vi "Shooter.vi"(8 "error in":errorcluster, 9 "Override?":bool, 10 "Override Setpoint":dbl, 11 "Load Ball Finished":bool) -> (0 "error out":errorcluster, 1 "Shooter Operation":T1(ring), 2 "Finished":bool, 3 "Load Ball":bool)   [LabVIEW 2015]
uses:
  <vilib>/Rock Robotics/WPI/CAN/TalonSRX/WPI_CANTalonSRX_APIControlMode.ctl
  <vilib>/Rock Robotics/Network Tables/NT Read Boolean.vi
  Robot Global Data.vi
  Team900-VIs/navX Library v2/navX Library v2.lvlib
panel:
  in  "Idle Speed":dbl=40.0 format="%#_13g"
  out "Shooter Speed (ticks per 100 ms)":dbl(graph)
  in  "Finished? (aim)":bool
  in  "Yaw":dbl
  out "SetSpeed":dbl
  in  "Goal Distance":dbl
  in  "Goal Angle":dbl
  in  "Goal Detected":bool
  in  "Distance to Motor Speed Conversions (Feet to ticks/100ms)":dbl[](array[numeric])=[250.0, 240.0, 210.0, 203.0, 193.0, 187.0, 192.0, 195.0, 197.0, 199.35, 201.73, 208.0]
  in  "Shooter Operation-Test Mode":T1(ring)
  in  "Encoder Velocity":dbl
  out "Turret Angle":T2(graph)
  in  "Setpoint":dbl format="%#_13g"
  in  "Speed Setpoint":dbl=220.0 format="%#_13g"
  in  "Max Shooter Speed (Rpm)":dbl=220.0
  in  "Turret revolutions per shooter revolution":dbl=15.0
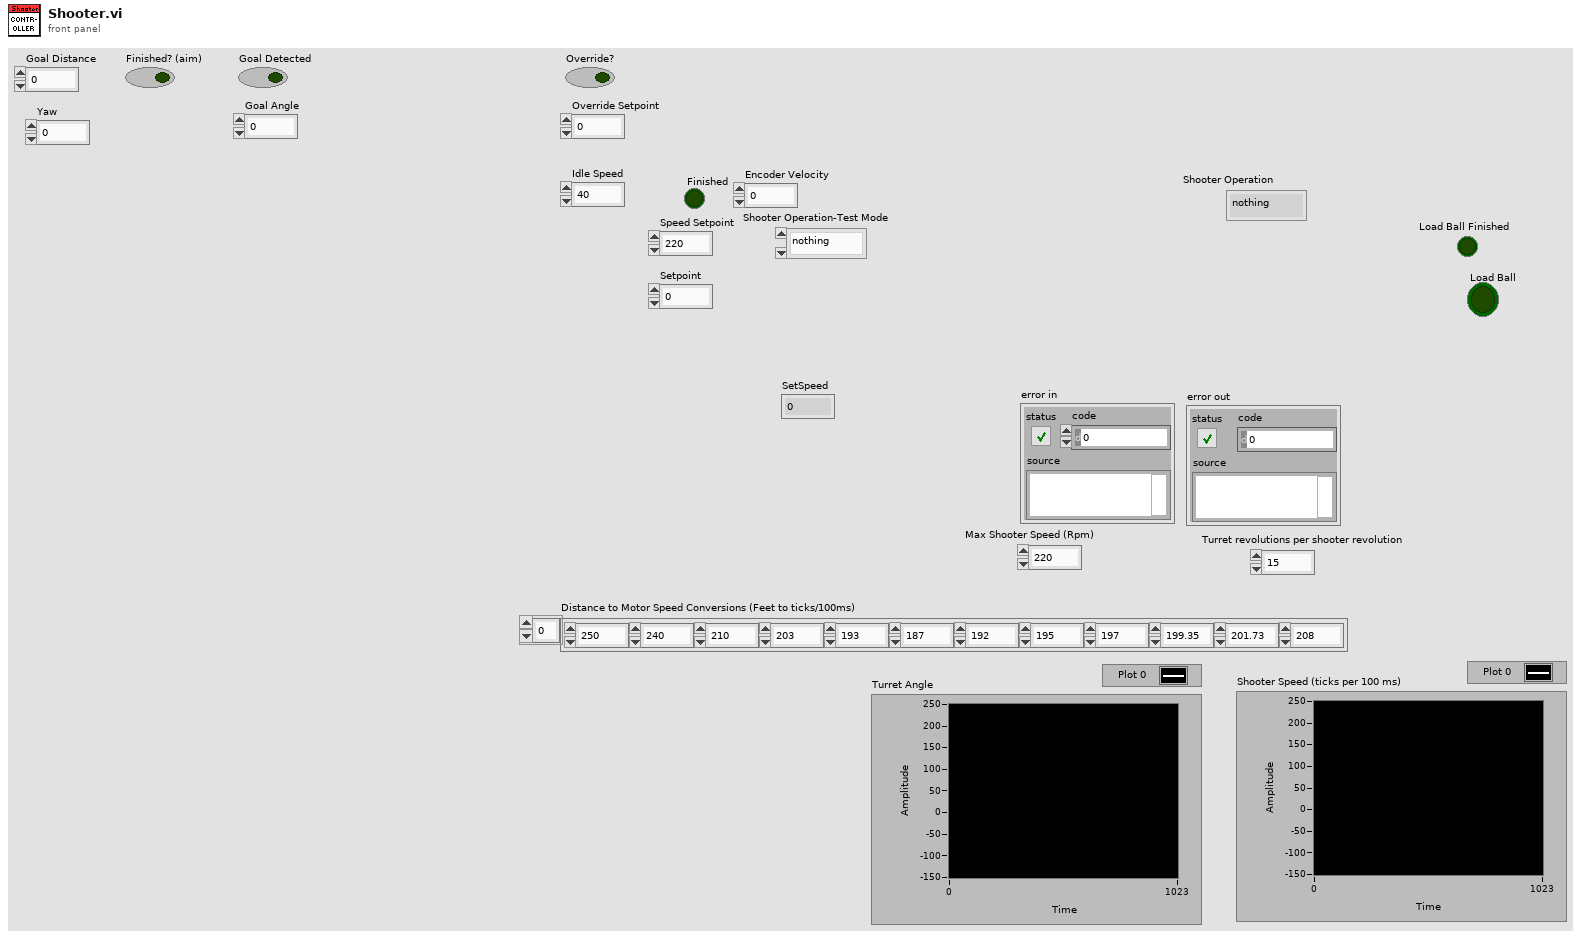
[diagram p1: front panel]
types:
  T1 = enum16{"nothing", "Fire", "Aim Goal", "Aim Foward"}
  T2 = cluster{"[0]":dbl, "[1]":dbl, "[2]":dbl, "[3]":dbl, "[4]":dbl, "[5]":dbl, "[6]":dbl, "[7]":dbl, "[8]":dbl}
  T3 = typedef "navX Library v2.lvlib/Z900_navX_DeviceTypeDef.ctl" = cluster{"Interface":cluster{"Protocol":T4, "Update Rate (4Hz-60Hz)":u8, "navX Open TypeDef":variant}, "Notify Packet":refnum<notifier>, "Loop VI Refnum":refnum<vi>, "Ready to Close Occurrence Refnum":refnum<k4>}
  T4 = typedef "navX Library v2.lvlib/Z900_navX_ProtocolTypeDef.ctl" = enum16{"SERIAL", "I2C", "SPI"}
  T5 = typedef "WPI_CANTalonSRX_APIControlMode.ctl" = enum8{"Percent VBus", "Speed", "Position", "Slave", "Unchanged / Invalid", "Voltage Compensation", "Current", "Motion Profile"}
  T6 = cluster{"Yaw":dbl, "Roll":dbl, "Pitch":dbl, "Heading":dbl, "Fused Heading":dbl}
  T7 = typedef "WPI_MotorControlDeviceRef.ctl" = cluster{"DeviceStatus":errorcluster, "Type":T8, "PWM":cluster{"PWM Channel":T9, "DeadBand":T10}, "CAN":cluster{"Device Number":u8, "Control Mode":T11, "Semaphore":T12, "Max Vout":dbl, "TalonSRX Control Mode":T5}, "Invert":bool}
  T8 = typedef "WPI_MotorControlType.ctl" = enum16{"PWM", "CAN", "CANTalonSRX"}
  T9 = typedef "FPGA_DIOPWMChannel.ctl" = enum8{"PWM 0", "PWM 1", "PWM 2", "PWM 3", "PWM 4", "PWM 5", "PWM 6", "PWM 7", "PWM 8", "PWM 9", "PWM MXP 0", "PWM MXP 1", "PWM MXP 2", "PWM MXP 3", "PWM MXP 4", "PWM MXP 5", "PWM MXP 6", "PWM MXP 7", "PWM MXP 8", "PWM MXP 9", "Invalid"}
  T10 = typedef "WPI_PWMDeadband.ctl" = cluster{"Name":string, "maxPositivePwm":i32, "minPositivePwm":i32, "centerPwm":i32, "maxNegativePwm":i32, "minNegativePwm":i32, "angularRange":u16}
  T11 = typedef "WPI_CANJaguar_ControlMode.ctl" = enum8{"Percent VBus", "Current", "Speed", "Position", "Voltage"}
  T12 = typedef "Semaphore RefNum" = refnum<k1>
  T13 = typedef "WPI_CANTalonSRX_GlobalStatus.ctl" = cluster{"Applied Throttle":dbl, "Module Enabled":bool, "CAN Error":errorcluster, "Closed Loop Error":dbl, "Forward Limit Switch Closed":bool, "Reverse Limit Switch Closed":bool, "Sensor Position":dbl, "Sensor Velocity":dbl, "Current":dbl, "Sticky Fault - Over Temp":bool, "Sticky Fault - Under Voltage":bool, "Sticky Fault - Forward Limit":bool, "Sticky Fault - Reverse Limit":bool, "Sticky Fault - Forward Soft Limit":bool, "Sticky Fault - Reverse Soft Limit":bool, "Brake is Enabled":bool, "Encoder Position":dbl, "Encoder Velocity":dbl, "Encoder Index Count":dbl, "Encoder A Pin State":bool, "Encoder B Pin State":bool, "Encoder Index Pin State":bool, "Analog In":dbl, "Analog In Velocity":dbl, "Temperature (C)":dbl, "Battery Voltage":dbl, "Control 5 Is Supported":bool, "Current Profile Slot Select":dbl, "Pos Div 8":bool, "Vel Div 4":bool, "Pulse Width Position":i32, "Pulse Width Velocity":i32, "Pulse Width Rise To Rise (us)":i32, "Pulse Width Rise To Fall (us)":i32, "Mot Prof Active Is Under Run":bool, "Mot Prof Active Has Under Run":bool, "Mot Prof Active Is Last":bool, "Mot Prof Active Velocity Only":bool, "Mot Prof Active Is Valid":bool, "Mot Prof Buffer Is Full":bool, "Mot Prof Active Profile Slot Select":i32, "Mot Prof NextID":i32, "Mot Prof Count":i32, "Mot Prof Active Velocity":dbl, "Mot Prof Active Position":dbl, "Mot Prof Output Enable":i32}
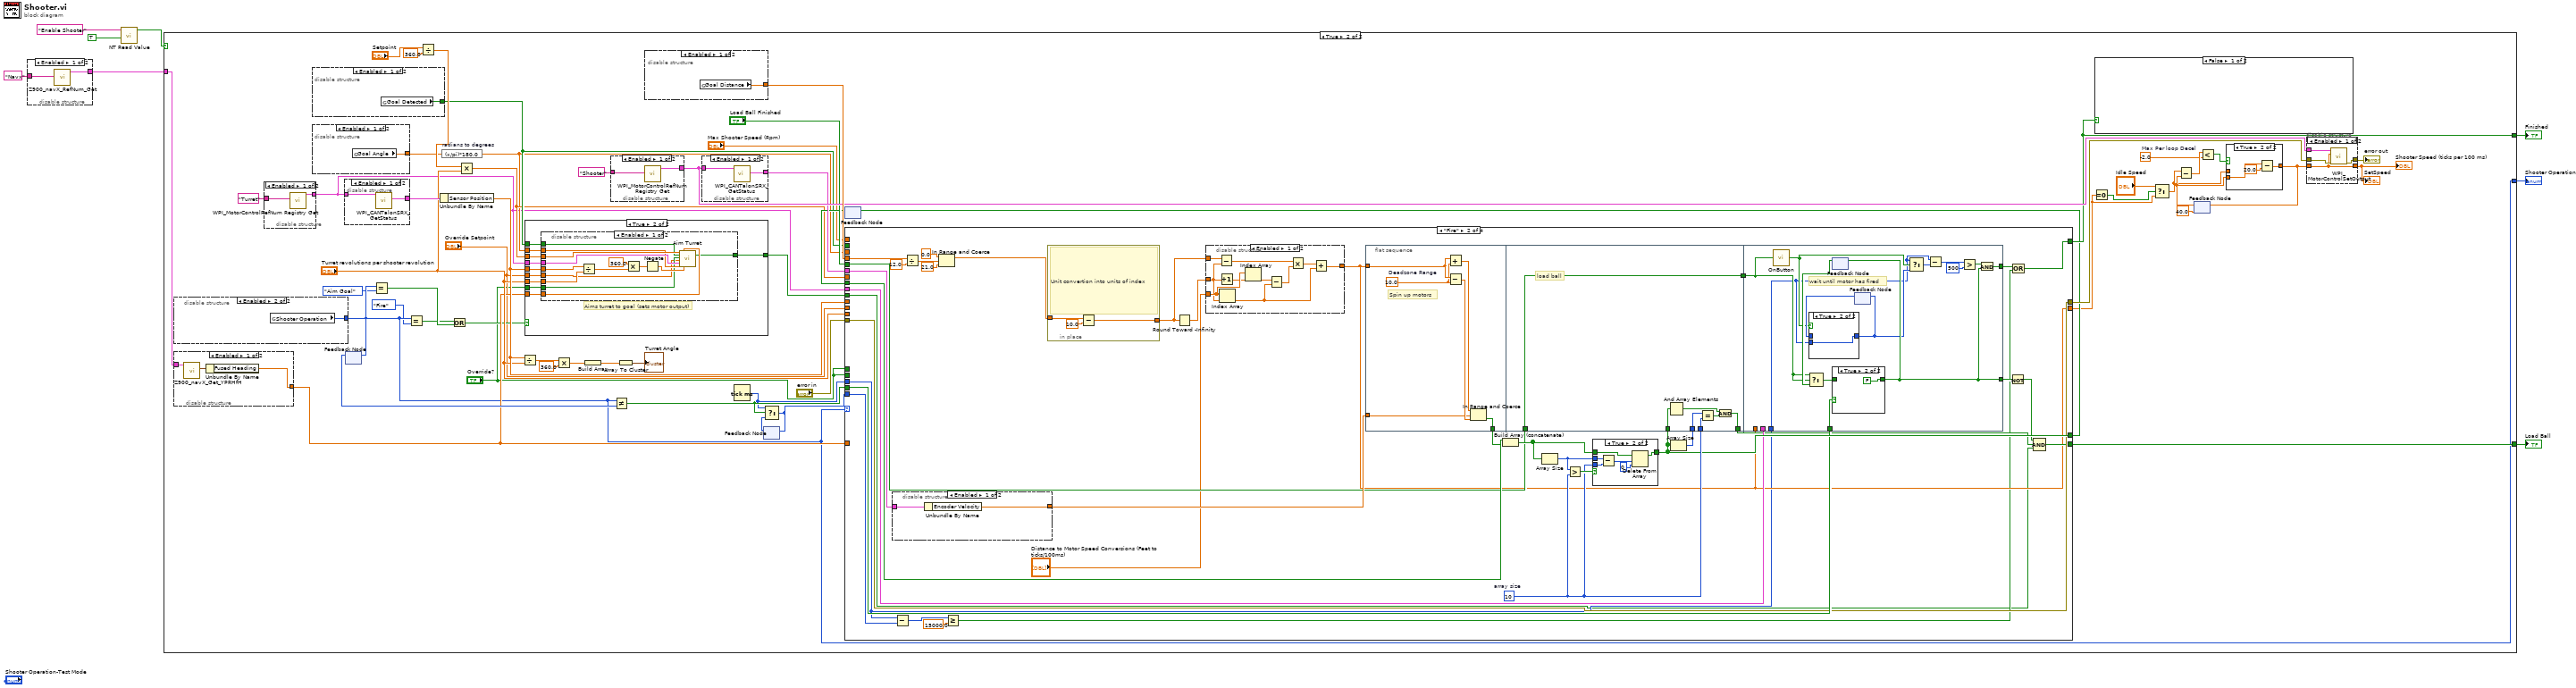
[diagram p0: block diagram]
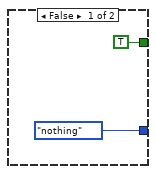
[diagram p3: hidden frame]
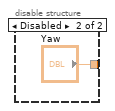
[diagram p5: hidden frame]
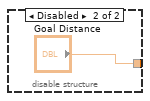
[diagram p6: hidden frame]
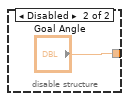
[diagram p7: hidden frame]
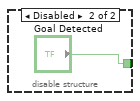
[diagram p8: hidden frame]
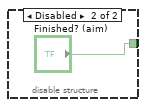
[diagram p10: hidden frame]
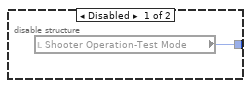
[diagram p11: hidden frame]
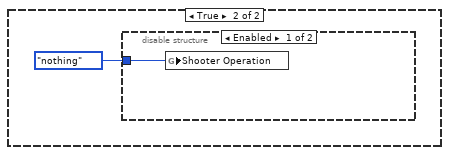
[diagram p17: hidden frame]
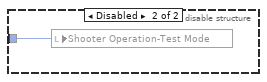
[diagram p18: hidden frame]
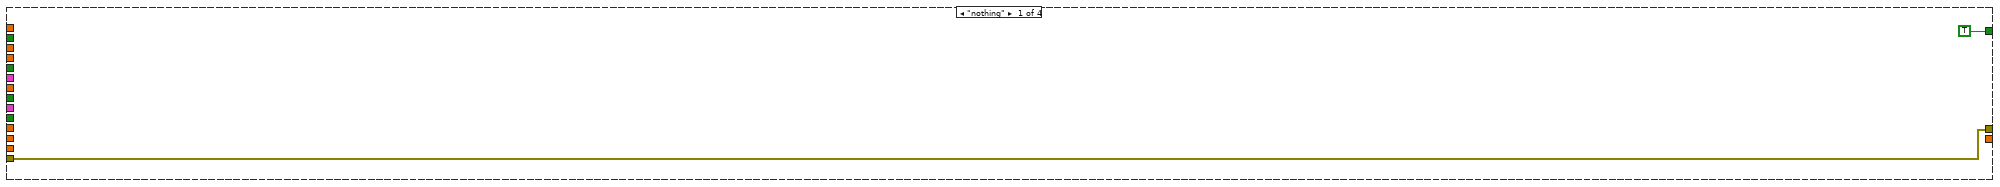
[diagram p19: hidden frame]
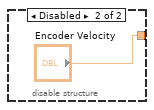
[diagram p20: hidden frame]
diagram:
  n1 = disable-structure shown="Enabled" {
    disable-tunnel: "Navx" ("refnum name") -> [w10 _]
    disable-tunnel: [w9 _] -> w1
    frame Enabled {
      n2 = call "Z900_navX_RefNum_Get.vi"("refnum name"=w10) -> ("navX Device"=w9:T3)  [unwired: 9 in, 1 out]
    }
    frame Disabled {
    }
  }
  n3 = call-poly <vilib>:"NT Read Value.vi"("Default Value"=TRUE, "Name"="Enable Shooter") -> ("Boolean"=w5:bool)  [unwired: 8 in, 1 out]
  n4 = case shown="True" w5 {
    tunnel: [_ w57] -> w6
    tunnel: [T1."nothing" ("Shooter Operation") w27] -> w8
    tunnel: [TRUE w55] -> w7
    tunnel: w1 -> [_ w41]
    frame False {
    }
    frame True {
      w21 = -2.0  # Max Per loop Decel
      n5 = disable-structure shown="Enabled" {
        disable-tunnel: [w109 w110] -> w27
        frame Disabled {
          n6 = local read "Shooter Operation-Test Mode"() -> (w109:T1)
        }
        frame Enabled {
          n7 = global read "Robot Global Data.vi" "Shooter Operation"() -> (w110:T1)
        }
      }
      n8 = disable-structure shown="Enabled" {
        disable-tunnel: w41 -> [w76 _]
        disable-tunnel: [w74 "Yaw"] -> w34
        frame Enabled {
          n9 = call "Z900_navX_Get_YPRHfH.vi"("navX Device"=w76) -> ("YRPHfH"=w75:T6)  [unwired: 7 in, 3 out]
          n10 = Unbundle By Name(w75) -> ("Fused Heading"=w74:dbl)
        }
        frame Disabled {
        }
      }
      n11 = disable-structure shown="Enabled" {
        disable-tunnel: "Turret" ("refnum name") -> [w116 _]
        disable-tunnel: [w115 _] -> w31
        frame Enabled {
          n12 = call <vilib>:"WPI_MotorControlRefNum Registry Get.vi"("refnum name"=w116) -> ("MotorControlDevRef"=w115:T7)  [unwired: 9 in, 1 out]
        }
        frame Disabled {
        }
      }
      n13 = disable-structure shown="Enabled" {
        disable-tunnel: [w82 "Goal Detected"] -> w42
        frame Enabled {
          n14 = global read "Robot Global Data.vi" "Goal Detected"() -> (w82:bool)
        }
        frame Disabled {
        }
      }
      n15 = disable-structure shown="Enabled" {
        disable-tunnel: [w80 "Goal Angle"] -> w23
        frame Enabled {
          n16 = global read "Robot Global Data.vi" "Goal Angle"() -> (w80:dbl)
        }
        frame Disabled {
        }
      }
      n17 = disable-structure shown="Enabled" {
        disable-tunnel: [w112 _] -> w51
        disable-tunnel: w31 -> [w111 _]
        frame Enabled {
          n18 = call <vilib>:"WPI_CANTalonSRX_GetStatus.vi"("CAN Talon SRX Ref"=w111) -> ("Talon SRX Status"=w112:T13)  [unwired: 8 in, 2 out]
        }
        frame Disabled {
        }
      }
      n19 = feedback #1() -> (w66:T1)  [unwired: 1 in]
      n20 = feedback-in #1(w27) -> ()
      n21 = Equal?(x=w27, y=T1."Aim Goal") -> (x = y?=w29:bool)
      n22 = Equal?(x=w27, y=T1."Fire") -> (x = y?=w28:bool)
      n23 = Divide(x="Setpoint", y=360.0) -> (x/y=w46:dbl)
      n24 = Unbundle By Name(w51) -> ("Sensor Position"=w36:dbl)
      n25 = expression code="(x/pi)*180.0" "radians to degrees"(w23) -> (w32:dbl)
      n26 = Or(x=w28, y=w29) -> (x .or. y?=w24:bool)
      n27 = Multiply(x=w46, y="Turret revolutions per shooter revolution") -> (x*y=w33:dbl)
      n28 = Divide(x=w36, y="Turret revolutions per shooter revolution") -> (x/y=w48:dbl)
      n29 = case shown="True" w24 {
        tunnel: w36 -> [_ w93]
        tunnel: "Turret revolutions per shooter revolution" -> [_ w92]
        tunnel: w34 -> [_ w91]
        tunnel: w33 -> [_ w90]
        tunnel: w32 -> [_ w89]
        tunnel: w31 -> [_ w88]
        tunnel: w42 -> [_ w87]
        tunnel: [_ w86] -> w30
        tunnel: "Override?" -> [_ w85]
        tunnel: "Override Setpoint" -> [_ w84]
        frame False {
        }
        frame True {
          # "Aims turret to goal (sets motor output)"
          n30 = disable-structure shown="Enabled" {
            disable-tunnel: w93 -> [w104 _]
            disable-tunnel: w92 -> [w103 _]
            disable-tunnel: w91 -> [w102 _]
            disable-tunnel: w90 -> [w101 _]
            disable-tunnel: w89 -> [w98 _]
            disable-tunnel: w88 -> [w99 _]
            disable-tunnel: w87 -> [w100 _]
            disable-tunnel: [w96 "Finished? (aim)"] -> w86
            disable-tunnel: w85 -> [w95 _]
            disable-tunnel: w84 -> [w94 _]
            frame Enabled {
              n31 = Divide(x=w104, y=w103) -> (x/y=w107:dbl)
              n32 = Multiply(x=360.0, y=w107) -> (x*y=w106:dbl)
              n33 = Negate(x=w106) -> (-x=w97:dbl)
              n34 = call "Aim Turret.vi"("Setpoint (testing purposes only)"=w101, "Goal Detected"=w100, "Override?"=w95, "Override Setpoint"=w94, "MotorControlDevRef"=w99, "Goal Angle Degrees 0=straight ahead"=w98, "Yaw (degrees 0 = straight ahead gets larger clockwise)"=w102, "Sensor Position (degrees)"=w97) -> ("Finished?"=w96:bool)  [unwired: 10 in, 1 out]
            }
            frame Disabled {
            }
          }
        }
      }
      n35 = Multiply(x=w48, y=360.0) -> (x*y=w44:dbl)
      n36 = Build Array(w44) -> (w50:dbl[])
      n37 = disable-structure shown="Enabled" {
        disable-tunnel: "Shooter" ("refnum name") -> [w118 _]
        disable-tunnel: [w117 _] -> w61
        frame Enabled {
          n38 = call <vilib>:"WPI_MotorControlRefNum Registry Get.vi"("refnum name"=w118) -> ("MotorControlDevRef"=w117:T7)  [unwired: 9 in, 1 out]
        }
        frame Disabled {
        }
      }
      n39 = Not Equal?(x=w27, y=w66) -> (x != y?=w52:bool)
      n40 = Array To Cluster(array=w50) -> (cluster=→"Turret Angle":T2)
      n41 = disable-structure shown="Enabled" {
        disable-tunnel: [w78 "Goal Distance"] -> w68
        frame Enabled {
          n42 = global read "Robot Global Data.vi" "Goal Distance"() -> (w78:dbl)
        }
        frame Disabled {
        }
      }
      n43 = disable-structure shown="Enabled" {
        disable-tunnel: w61 -> [w114 _]
        disable-tunnel: [w113 _] -> w58
        frame Enabled {
          n44 = call <vilib>:"WPI_CANTalonSRX_GetStatus.vi"("CAN Talon SRX Ref"=w114) -> ("Talon SRX Status"=w113:T13)  [unwired: 8 in, 2 out]
        }
        frame Disabled {
        }
      }
      n45 = Tick Count (ms)() -> (millisecond timer value=w37:u32)
      n46 = feedback #2() -> (w65:u32)  [unwired: 1 in]
      n47 = Select(t=w37, s=w52, f=w65) -> (s? t:f=w64:u32)
      n48 = feedback-in #2(w64) -> ()
      n49 = feedback #3() -> (w54:bool[])  [unwired: 1 in]
      n50 = case shown="\"Fire\"" w27 {
        tunnel: [TRUE w156 w222 w227] -> w55
        tunnel: w32 -> [_ _ _ _]
        tunnel: w68 -> [_ w134 _ _]
        tunnel: [_ w140 _ _] -> w40
        tunnel: w58 -> [_ w166 _ _]
        tunnel: w54 -> [_ w163 _ _]
        tunnel: "error in" -> [w129 w149 w223 w231]
        tunnel: w42 -> [_ _ _ _]
        tunnel: w31 -> [_ w146 _ w232]
        tunnel: "Max Shooter Speed (Rpm)" -> [_ _ _ _]
        tunnel: w34 -> [_ _ _ _]
        tunnel: w64 -> [_ w153 _ _]
        tunnel: [w129 w149 w223 w238] -> w60
        tunnel: [_ w143 _ _] -> w57
        tunnel: "Load Ball Finished" -> [_ w148 _ _]
        tunnel: [_ w152 _ _] -> w53
        tunnel: w37 -> [_ w138 _ _]
        tunnel: w52 -> [_ w150 _ _]
        tunnel: w33 -> [_ _ _ w237]
        tunnel: "Turret revolutions per shooter revolution" -> [_ _ _ w229]
        tunnel: w36 -> [_ _ _ w230]
        tunnel: w30 -> [_ w135 w222 _]
        tunnel: "Override Setpoint" -> [_ _ _ w226]
        tunnel: "Override?" -> [_ _ _ w225]
        tunnel: "Override?" -> [_ _ _ w224]
        frame "nothing" {
        }
        frame "Fire" {
          w158 = 10  # array size
          n51 = disable-structure shown="Enabled" {
            disable-tunnel: w166 -> [w168 _]
            disable-tunnel: [w167 "Encoder Velocity"] -> w165
            frame Enabled {
              n52 = Unbundle By Name(w168) -> ("Encoder Velocity"=w167:dbl)
            }
            frame Disabled {
            }
          }
          n53 = Subtract(x=w138, y=w153) -> (x-y=w154:u32)
          n54 = Divide(x=w134, y=12.0) -> (x/y=w133:dbl)
          n55 = In Range and Coerce(upper limit=0.0, x=w133, lower limit=21.0) -> (coerced(x)=w130:dbl)  [unwired: 1 out]
          n56 = Greater Or Equal?(x=w154, y=15000.0) -> (x >= y?=w139:bool)
          n57 = in-place {
            in-place-border: [w171] -> w141
            in-place-border: w130 -> [w172]
            # "Unit convertion into units of index"
            n58 = Subtract(x=w172, y=10.0) -> (x-y=w171:dbl)
          }
          n59 = Round Toward -Infinity(1:w141) -> (0:w142:dbl)
          n60 = disable-structure shown="Enabled" {
            disable-tunnel: "Distance to Motor Speed Conversions (Feet to ticks/100ms)" -> [w182 _]
            disable-tunnel: [w175 "Speed Setpoint"] -> w140
            disable-tunnel: w142 -> [w174 _]
            disable-tunnel: w141 -> [w173 _]
            frame Enabled {
              n61 = Subtract(x=w173, y=w174) -> (x-y=w176:dbl)
              n62 = Increment(x=w174) -> (x+1=w181:dbl)
              n63 = Index Array(array=w182, index=w174) -> (element=w178:dbl)
              n64 = Index Array(array=w182, index=w181) -> (element=w180:dbl)
              n65 = Subtract(x=w180, y=w178) -> (x-y=w179:dbl)
              n66 = Multiply(x=w176, y=w179) -> (x*y=w177:dbl)
              n67 = Add(x=w177, y=w178) -> (x+y=w175:dbl)
            }
            frame Disabled {
            }
          }
          n68 = flat-sequence {
            tunnel: w140 -> [w192]
            tunnel: w165 -> [w193]
            tunnel: [w194] -> w162
            tunnel: [w200] -> w164
            tunnel: w152 -> [w201]
            tunnel: w158 -> [w203]
            tunnel: w157 -> [w202]
            tunnel: [w197] -> w144
            tunnel: w148 -> [w200]
            tunnel: w164 -> [w208]
            tunnel: w146 -> [_]
            tunnel: w140 -> [_]
            tunnel: w138 -> [w204]
            tunnel: [w212] -> w151
            tunnel: w150 -> [w210]
            tunnel: [w209] -> w147
            frame #0 {
              w191 = 10.0  # Deadzone Range
              # "Spin up motors"
              n69 = Add(x=w192, y=w191) -> (x+y=w195:dbl)
              n70 = Subtract(x=w192, y=w191) -> (x-y=w196:dbl)
              n71 = In Range and Coerce(upper limit=w195, x=w193, lower limit=w196) -> (In Range?=w194:bool)  [unwired: 1 out]
            }
            frame #1 {
              # "load ball"
              n72 = And Array Elements(Boolean array=w201) -> (logical AND=w198:bool)
              n73 = Equal?(x=w202, y=w203) -> (x = y?=w199:bool)
              n74 = And(x=w198, y=w199) -> (x .and. y?=w197:bool)
            }
            frame #2 {
              # "wait until motor has fired"
              n75 = call "OnButton.vi"("Button"=w208) -> ("Value"=w207:bool)  [unwired: 1 in]
              n76 = feedback #4() -> (w211:bool)  [unwired: 1 in]
              n77 = Select(t=w208, s=w208, f=w211) -> (s? t:f=w217:bool)
              n78 = case shown="True" w210 {
                tunnel: [w218 FALSE] -> w209
                tunnel: w217 -> [w218 _]
                frame False {
                }
                frame True {
                }
              }
              n79 = feedback-in #4(w209) -> ()
              n80 = feedback #5() -> (w216:u32)  [unwired: 1 in]
              n81 = case shown="True" w207 {
                tunnel: [w220 w221] -> w206
                tunnel: w204 -> [_ w221]
                tunnel: w216 -> [w220 _]
                frame False {
                }
                frame True {
                }
              }
              n82 = feedback-in #5(w206) -> ()
              n83 = Select(t=w204, s=w207, f=w206) -> (s? t:f=w205:u32)
              n84 = Subtract(x=w204, y=w205) -> (x-y=w215:u32)
              n85 = Greater?(x=w215, y=500) -> (0:w213:bool)
              n86 = And(x=w213, y=w209) -> (x .and. y?=w212:bool)
            }
          }
          n87 = Build Array (concatenate)(w163, w162) -> (w160:bool[])
          n88 = Array Size(array=w160) -> (size(s)=w159:i32)
          n89 = Greater?(x=w159, y=w158) -> (0:w161:bool)
          n90 = case shown="True" w161 {
            tunnel: w160 -> [w184 w190]
            tunnel: w158 -> [_ w189]
            tunnel: w159 -> [_ w188]
            tunnel: [w184 w187] -> w152
            frame False {
            }
            frame True {
              n91 = Subtract(x=w188, y=w189) -> (x-y=w186:i32)
              n92 = Delete From Array(array=w190, length=w186, index=0) -> (array with subset deleted=w187:bool[])  [unwired: 1 out]
            }
          }
          n93 = Array Size(array=w152) -> (size(s)=w157:i32)
          n94 = Not(x=w147) -> (.not. x?=w145:bool)
          n95 = Compound Arithmetic op=OR(w151, w139) -> (w156:bool)
          n96 = Compound Arithmetic op=AND(w145, w144, w135) -> (w143:bool)
        }
        frame "Aim Goal" {
        }
        frame "Aim Foward" {
          w234 = 0.0  # Value when turrent is facing straight ahead (-225 to 225)
          w228 = 0.35  # Angle Tolerance
          n97 = Divide(x=w230, y=w229) -> (x/y=w236:dbl)
          n98 = Negate(x=w228) -> (-x=w239:dbl)
          n99 = Multiply(x=w236, y=360.0) -> (x*y=w233:dbl)
          n100 = In Range and Coerce(upper limit=w228, x=w233, lower limit=w239) -> (In Range?=w227:bool)  [unwired: 1 out]
          n101 = disable-structure shown="Enabled" {
            disable-tunnel: w234 -> [w241 _ _]
            disable-tunnel: w232 -> [w245 w261 _]
            disable-tunnel: w231 -> [w243 _ w263]
            disable-tunnel: [w242 _ w263] -> w238
            disable-tunnel: w237 -> [_ w262 _]
            disable-tunnel: w226 -> [w244 _ _]
            disable-tunnel: w225 -> [_ _ _]
            disable-tunnel: w224 -> [w240 _ _]
            frame Enabled {
              n102 = case shown="False" w240 {
                tunnel: w245 -> [w251 w259]
                tunnel: w244 -> [_ w260]
                tunnel: w243 -> [w249 w256]
                tunnel: [w247 w254] -> w242
                tunnel: w241 -> [w246 _]
                frame False {
                  n103 = call <vilib>:"WPI_CANTalonSRX_ChangeMode.vi"("error in (no error)"=w249, "Control Mode"=WPI_CANTalonSRX_APIControlMode."Position", "CAN Talon SRX Ref"=w251) -> ("error out"=w248:errorcluster, "CAN Talon SRX Ref"=w250:T7)  [unwired: 7 in]
                  n104 = call <vilib>:"WPI_MotorControlSetOutput.vi"("error in (no error)"=w248, "Sync Group / Parameter Slot"=u8 0, "Output"=w246, "MotorControlDevRef"=w250) -> ("error out"=w247:errorcluster)  [unwired: 5 in, 2 out]
                }
                frame True {
                  n105 = call <vilib>:"WPI_CANTalonSRX_ChangeMode.vi"("error in (no error)"=w256, "Control Mode"=WPI_CANTalonSRX_APIControlMode."Percent VBus", "CAN Talon SRX Ref"=w259) -> ("error out"=w255:errorcluster, "CAN Talon SRX Ref"=w258:T7)  [unwired: 7 in]
                  n106 = call <vilib>:"WPI_MotorControlSetOutput.vi"("error in (no error)"=w255, "Output"=w260, "MotorControlDevRef"=w258) -> ("error out"=w254:errorcluster)  [unwired: 6 in, 2 out]
                }
              }
            }
            frame Disabled {
              n107 = call <vilib>:"WPI_MotorControlSetOutput.vi"("Output"=w262, "MotorControlDevRef"=w261) -> ()  [unwired: 7 in, 3 out]
            }
            frame Disabled {
            }
          }
        }
      }
      n108 = feedback-in #3(w53) -> ()
      n109 = Equal To 0?(x=w40) -> (x = 0?=w62:bool)
      n110 = case shown="False" w55 {
        frame False {
        }
        frame True {
          n111 = disable-structure shown="Enabled" {
            disable-tunnel: T1."nothing" ("Shooter Operation") -> [w126 w127]
            frame Enabled {
              n112 = global write "Robot Global Data.vi" "Shooter Operation"(w126) -> ()
            }
            frame Disabled {
              n113 = local write "Shooter Operation-Test Mode"(w127) -> ()
            }
          }
        }
      }
      n114 = Select(t="Idle Speed", s=w62, f=w40) -> (s? t:f=w17:dbl)
      n115 = feedback #6(40.0 ("Idle Speed")) -> (w19:dbl)
      n116 = Subtract(x=w17, y=w19) -> (x-y=w22:dbl)
      n117 = Less?(x=w22, y=w21) -> (x < y?=w20:bool)
      n118 = case shown="True" w20 {
        tunnel: w19 -> [_ w73]
        tunnel: [w70 w71] -> w18
        tunnel: w17 -> [w70 _]
        frame False {
        }
        frame True {
          n119 = Subtract(x=w73, y=20.0) -> (x-y=w71:dbl)
        }
      }
      n120 = feedback-in #6(w18) -> ()
      n121 = disable-structure shown="Enabled" {
        disable-tunnel: w61 -> [w122 _]
        disable-tunnel: w18 -> [w119 w123]
        disable-tunnel: w60 -> [w121 w124]
        disable-tunnel: [w120 w124] -> w59
        disable-tunnel: [w119 w123] -> w13
        frame Enabled {
          n122 = call <vilib>:"WPI_MotorControlSetOutput.vi"("error in (no error)"=w121, "Output"=w119, "MotorControlDevRef"=w122) -> ("error out"=w120:errorcluster)  [unwired: 6 in, 2 out]
        }
        frame Disabled {
        }
      }
      "error out" <- w59
      "SetSpeed" <- w13
      "Shooter Speed (ticks per 100 ms)" <- w13
    }
  }
  "Load Ball" <- w6
  "Shooter Operation" <- w8
  "Finished" <- w7
